vi "Update Data.vi"(8 "error in (no error)":errorcluster, 9 "data":waveform(dbl)[](array[waveform]), 10 "Channel Names":string[](array[string]), 11 "Table View in":refnum<class "Table View.lvclass">) -> (0 "error out":errorcluster, 3 "Table View out":refnum<class "Table View.lvclass">)   [LabVIEW 2020, in "[V]Table View.lvlib" / "Table View.lvclass"]
uses:
  Table View.lvclass
  <vilib>/HUASUI/MulListBox/Type Definitions/Autosize Mode.ctl
  Table View.lvclass/Table View.ctl
  <vilib>/HUASUI/MulListBox/MListBox.lvclass/MListBox.ctl
  <vilib>/Waveform/WDTOps.llb/WDT Get Waveform Time Array DBL.vi
  <vilib>/HUASUI/MulListBox/MListBox.lvclass
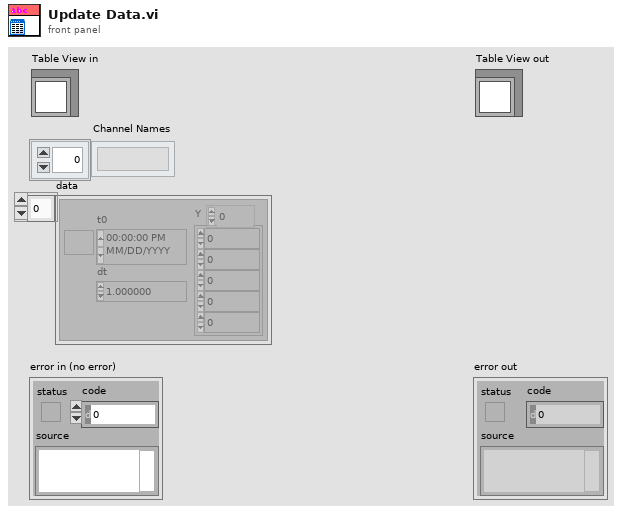
[diagram p1: front panel]
types:
  T1 = typedef "Autosize Mode.ctl" = enum16{"Header", "All Cells"}
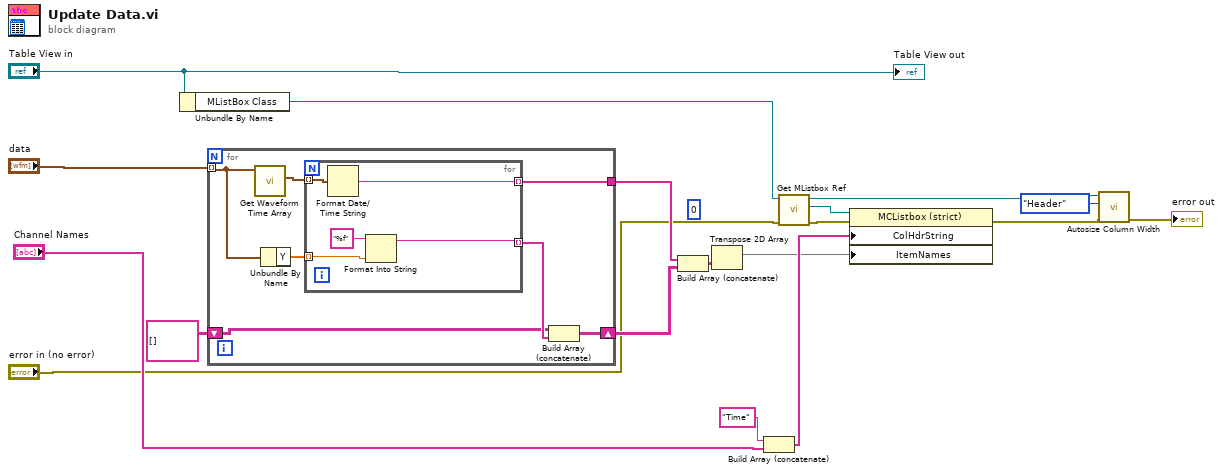
[diagram p0: block diagram]
diagram:
  (unwired) i16 0 ("Index")
  n1 = Unbundle By Name("Table View in") -> ("MListBox Class"=w2:refnum<class "MListBox.lvclass">)
  n2 = for {
    tunnel: "data" -> [w25] mode=indexing
    tunnel: [w22] -> w11
    shift-right: [w21] -> w4
    shift-left: string[][] [] -> [w19]
    n3 = call-poly <vilib>:"Get Waveform Time Array.vi"("waveform in"=w25) -> ("X array"=w24:timestamp[])  [unwired: 9 in, 1 out]
    n4 = Unbundle By Name(w25) -> ("Y"=w23:dbl[])
    n5 = for {
      tunnel: w24 -> [w30] mode=indexing
      tunnel: w23 -> [w28] mode=indexing
      tunnel: [w27] -> w22 mode=indexing
      tunnel: [w26] -> w20 mode=indexing
      n6 = Format Date/Time String(seconds (now)=w30) -> (date/time string=w27:string)  [unwired: 2 in]
      n7 = Format Into String(format string="%f", w28) -> (resulting string=w26:string)  [unwired: 2 in, 1 out]
    }
    n8 = Build Array (concatenate)(w19, w20) -> (w21:string[][])
  }
  n9 = Build Array (concatenate)(w11, w4) -> (w6:string[][])
  n10 = Transpose 2D Array(2D array=w6) -> (transposed array=w1:string[][])
  n11 = Build Array (concatenate)("Time", "Channel Names") -> (w13:string[])
  n12 = call <vilib>:"Get MListbox Ref.vi"("error in (no error)"="error in (no error)", "Multicolumn ListBox in"=w2) -> ("error out"=w12:errorcluster, "MListbox Ref"=w14:refnum<vi>, "Multicolumn ListBox out"=w9:refnum<class "MListBox.lvclass">)  [unwired: 7 in]
  n13 = property class="MCListbox (strict)"(reference=w14, error in=w12, "ColHdrString"=w13, "ItemNames"=w1) -> (error out=w8:errorcluster)  [unwired: 1 out]
  n14 = call <vilib>:"Autosize Column Width.vi"("error in (no error)"=w8, "Autosize Mode"=Autosize_Mode."Header", "Multicolumn ListBox in"=w9) -> ("error out"=→"error out":errorcluster)  [unwired: 7 in, 1 out]
  "Table View out" <- "Table View in"
